vi "Keithley 2400 - VoltSource.vi"(10 "Tensão aplicada:":dbl=10.0, 11 "Porta:":refnum<visa-resource-name>="COM5") -> (0 "Corrente:":dbl, 3 "Tensão:":dbl)   [LabVIEW 2018]
uses:
  <vilib>/Instr/_visa.llb/VISA Configure Serial Port (Instr).vi
panel:
  out "error out":errorcluster
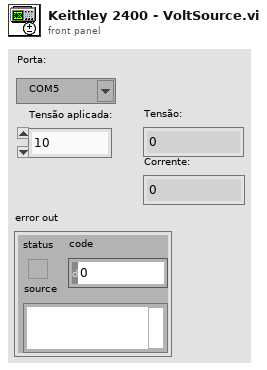
[diagram p1: front panel]
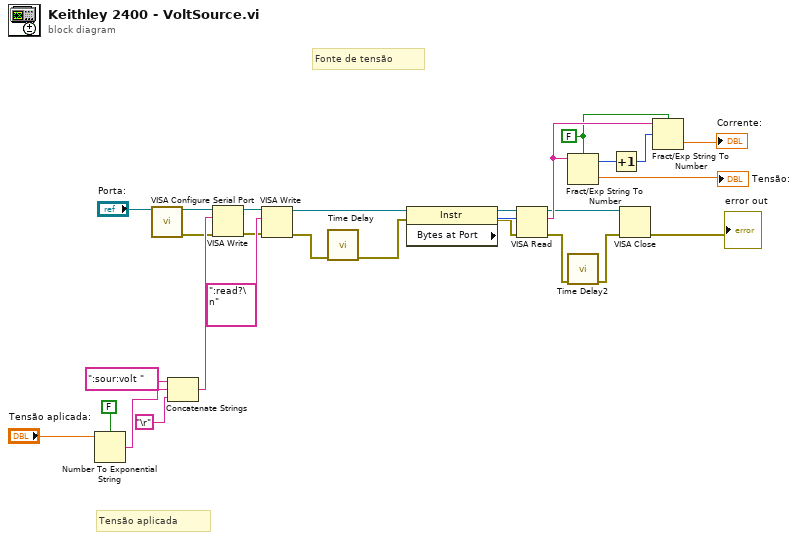
[diagram p0: block diagram]
diagram:
  w9 = FALSE ("use system decimal point (T)")
  # "Tensão aplicada"
  # "Fonte de tensão"
  n1 = Number To Exponential String(number="Tensão aplicada:", 1:FALSE ("use system decimal point (T)")) -> (E-format string=w8:string)  [unwired: 2 in]
  n2 = call-poly "VISA Configure Serial Port"("VISA resource name"="Porta:") -> ("VISA resource name out"=w4:refnum<visa-resource-name>, "error out"=w3:errorcluster)  [unwired: 13 in]
  n3 = Concatenate Strings(":sour:volt " ("string"), w8, "\r") -> (w26:string)
  n4 = VISA Write(VISA resource name=w4, write buffer=w26, error in (no error)=w3) -> (VISA resource name out=w22:refnum<visa-resource-name>, error out=w23:errorcluster)  [unwired: 1 out]
  n5 = VISA Write(VISA resource name=w22, write buffer=":read?\n", error in (no error)=w23) -> (VISA resource name out=w20:refnum<visa-resource-name>, error out=w24:errorcluster)  [unwired: 1 out]
  n6 = call "Time Delay"("error in (no error)"=w24) -> ("error out"=w21:errorcluster)  [unwired: 10 in]
  n7 = property class="Instr"(reference=w20, error in=w21) -> (reference out=w18:refnum<visa-resource-name>, error out=w17:errorcluster, "Bytes at Port"=w19:u32)
  n8 = VISA Read(VISA resource name=w18, byte count=w19, error in (no error)=w17) -> (VISA resource name out=w5:refnum<visa-resource-name>, read buffer=w14:string, error out=w2:errorcluster)  [unwired: 1 out]
  n9 = Fract/Exp String To Number(use system decimal point (T)=w9, string=w14) -> (offset past number=w13:i32, number=→"Tensão:":dbl)  [unwired: 2 in]
  n10 = call "Time Delay2"("error in (no error)"=w2) -> ("error out"=w1:errorcluster)  [unwired: 10 in]
  n11 = Increment(x=w13) -> (x+1=w12:i32)
  n12 = VISA Close(VISA resource name=w5, error in (no error)=w1) -> (error out=→"error out":errorcluster)
  n13 = Fract/Exp String To Number(use system decimal point (T)=w9, string=w14, offset=w12) -> (number=→"Corrente:":dbl)  [unwired: 1 in, 1 out]
